vi "Error state.vi"(8 "error in (no error)":errorcluster, 11 "Nested in":refnum<class "Nested.lvclass">) -> (0 "error out":errorcluster, 3 "Nested out":refnum<class "Nested.lvclass">)   [LabVIEW 2020, in "Nested.lvlib" / "Nested.lvclass"]
uses:
  Nested.lvclass
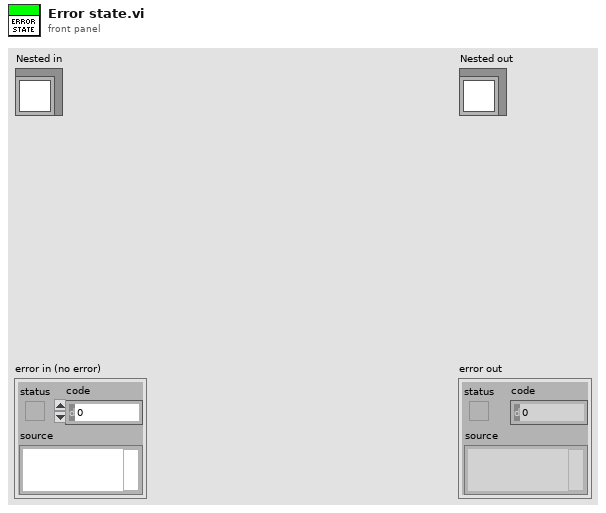
[diagram p1: front panel]
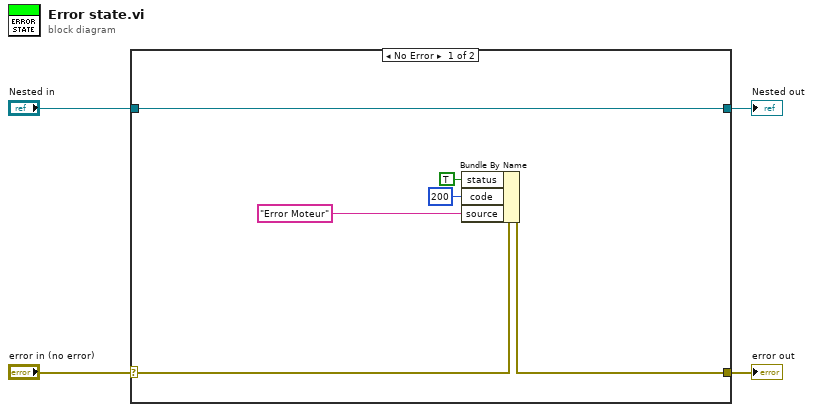
[diagram p0: block diagram]
diagram:
  n1 = case shown="No Error" "error in (no error)" {
    selector: "error in (no error)" -> [w9 w12]
    tunnel: [w8 w12] -> w3
    tunnel: [w10 w11] -> w1
    tunnel: "Nested in" -> [w10 w11]
    frame No Error {
      n2 = Bundle By Name(cluster=w9, "status"=TRUE, "code"=200, "source"="Error Moteur") -> (w8:errorcluster)
    }
    frame Error {
    }
  }
  "error out" <- w3
  "Nested out" <- w1
